vi "运维调试_氨氮.vi"() -> ()   [LabVIEW 2016, in "氨氮.lvlib"]
uses:
  <vilib>/Platform/TimedLoop/XDataNode/timing_clust.ctl
  <vilib>/Platform/TimedLoop/XDataNode/nitl_modes.ctl
  <vilib>/Platform/TimedLoop/XDataNode/wakeup.ctl
  <vilib>/Utility/miscctls.llb/LVPointTypeDef.ctl
  <vilib>/Platform/TimedLoop/XDataNode/XDataNode.xnode
  <vilib>/Platform/TimedLoop/XDataNode/XDNodeRunTimeDep.lvlib
  <vilib>/Utility/config.llb/NI_LVConfig.lvlib
panel:
  in  "氨氮自动测试量程配置":T1
  out "ADC":sgl
  out "温度2":sgl
  out "温度1":sgl
  out "固件版本号":string
  in  "数组":string[](array[string])
  in  "备用系数写入":bool
  in  "备用系数读取":bool
  in  "备用系数":T2
  in  "量程切换阈值写入":bool
  in  "量程切换阈值读取":bool
  in  "量程切换阈值":cluster{"阈值":dbl, "标液浓度":dbl}
  in  "参数下拉列表":enum16{"氨氮", "总磷"}(ring)
  in  "量程下拉列表":enum16{"低量程", "高量程"}(ring)
  in  "测量模式下拉列表":enum16{"水样测量", "空白核查", "跨度核查", "标样核查", "加标回收"}(ring)
  in  "公式":cluster{"X^2":dbl, "X":dbl, "b":dbl}
  in  "写公式":bool
  in  "读公式":bool
  in  "精度":dbl=4.0
  in  "样品5 F0":dbl
  in  "样品5 F1":dbl
  in  "样品4 F1":dbl
  in  "样品4 F0":dbl
  in  "样品3 F0":dbl
  in  "样品3 F1":dbl
  in  "样品2 F0":dbl
  in  "样品2 F1":dbl
  in  "样品1 F1":dbl
  in  "样品1 F0":dbl
  in  "method":u16(ring) items=["最小二乘", "最小绝对残差", "Bisquare"]
  in  "模型":enum32{"线性", "多项式"}(ring)
  out "r^2":dbl format="%.7g"
  out "拟合公式":string
  in  "样品2启用":bool
  in  "样品5启用":bool
  in  "样品4启用":bool
  in  "样品3启用":bool
  in  "样品1启用":bool
  in  "标液浓度5":dbl
  out "测量吸光度5":dbl
  in  "标液浓度4":dbl
  out "测量吸光度4":dbl
  in  "标液浓度3":dbl
  out "测量吸光度3":dbl
  in  "标液浓度2":dbl
  out "测量吸光度2":dbl
  out "测量吸光度1":dbl
  in  "标液浓度1":dbl
  out "XY图":cluster{"X Values":dbl[], "Y Values":dbl[]}[](graph)
  in  "返回":bool
  in  "设置":bool
  out "序列号":string="序列号"
  out "氨氮测量数据":T3(xcontrol)
  out "集成报警信息":string
  out "设置值":dbl
  out "定时启动":bool
  out "总磷总氮运行状态":T4(xcontrol)
  in  "停止":bool
  in  "手动启动":bool
  in  "单步测试":bool
  in  "总磷氨氮调试":u16[](xcontrol)
  out "F3":sgl format="%#.6f"
  out "F2":sgl format="%#.6f"
  out "F1":sgl format="%#.6f"
  out "F0":sgl format="%#.6f"
  out "多列列表框":i32(listbox)
  # "COM7"
  # "参数设置"
  # "标液浓度"
  # "F0"
  # "F1"
  # "吸光值显示"
  # "样品一"
  # "辅\n助\n计\n算\n区"
  # "样品二"
  # "样品三"
  # "样品四"
  # "样品五"
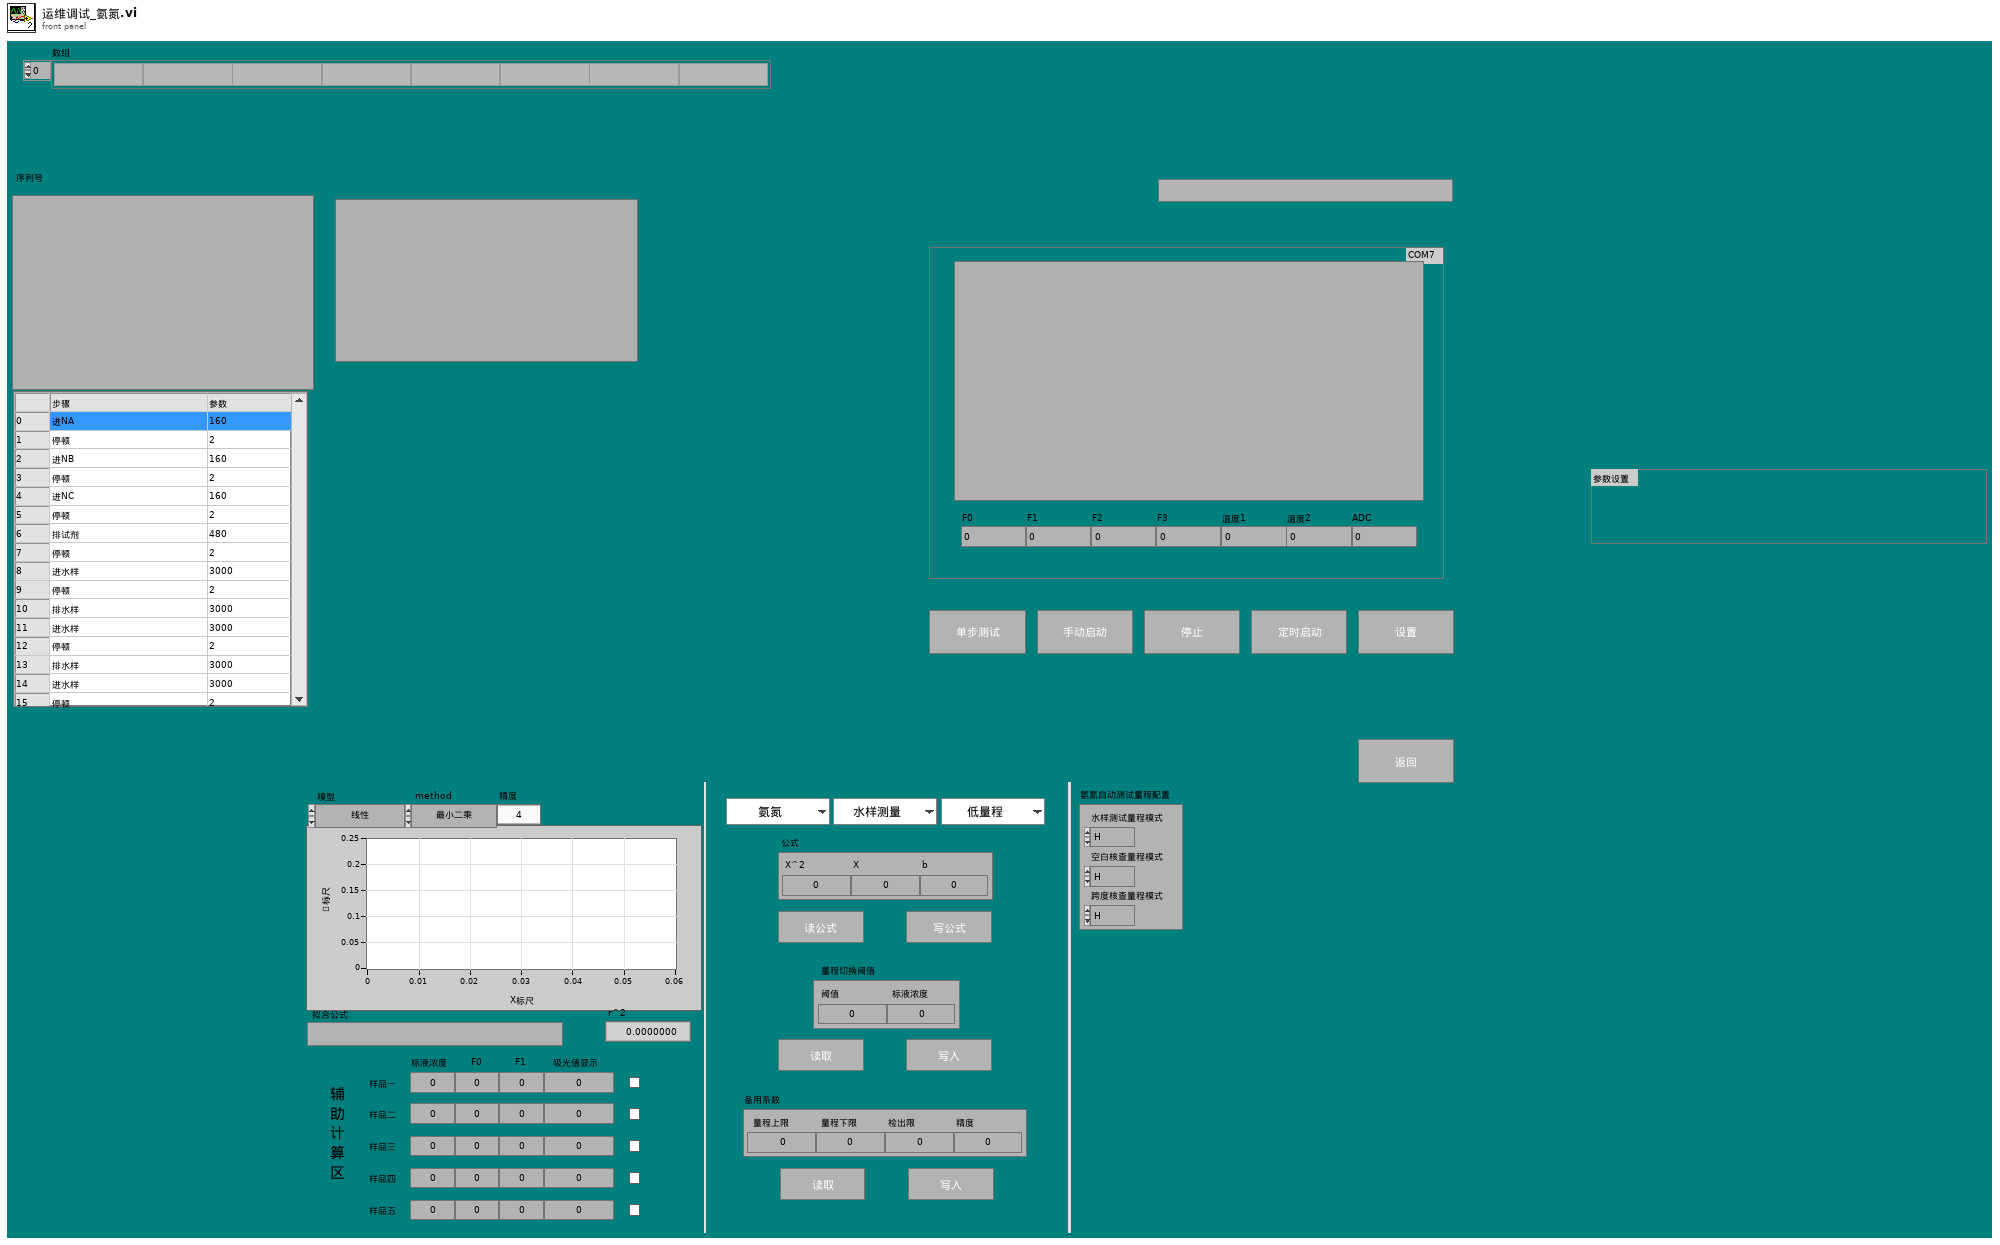
[diagram p1: front panel]
types:
  T1 = cluster{"水样测试量程模式":enum16{"H", "L", "AUTO"}, "空白核查量程模式":enum16{"H", "L", "AUTO"}, "跨度核查量程模式":enum16{"H", "L", "AUTO"}}
  T2 = cluster{"量程上限":dbl, "量程下限":dbl, "检出限":dbl, "精度":dbl}
  T3 = cluster{"flowid":u16, "测量精度":u16, "测量数据区":cluster{"因子编码":u32, "单位":u16, "标样参考值":sgl, "水样数据时间":timestamp, "水样实测值":sgl, "水样数据标识":string, "标样数据时间":timestamp, "标样实测值":sgl, "标样数据标识":string, "空白数据时间":timestamp, "空白实测值":sgl, "空白数据标识":string, "零点核查数据时间":timestamp, "零点核查实测值":sgl, "零点核查数据标识":string, "跨度核查数据时间":timestamp, "跨度核查实测值":sgl, "跨度核查数据标识":string, "加标回收数据时间":timestamp, "加标回收实测值":sgl, "加标回收数据标识":string, "平行样数据时间":timestamp, "平行样实测值":sgl, "平行样数据标识":string}}
  T4 = cluster{"系统时间":timestamp, "工作状态":enum16{"空闲", "水样测试", "标样核查", "零点核查", "跨度核查", "空白测试", "平行样测试", "加标回收", "空白校准", "标样校准", "初始化（清洗）"}, "测量模式":enum16{"待机", "连续模式", "周期模式", "定点模式", "受控模式", "手动模式"}, "告警代码":enum16{"无告警", "缺试剂告警", "缺水样告警", "缺蒸馏水告警", "缺标液告警", "仪表漏液告警", "标定异常告警", "超量程告警", "加热异常", "低试剂预警", "超上限告警", "超下限告警", "仪表内部其他异常", "滴定异常告警", "电极异常告警", "量程切换告警", "参数设置告警", "PH电极电位异常", "电导率电极异常", "浊度光度异常", "溶解氧电极异常", "溶解氧光强异常", "温度异常告警", "PH异常告警", "溶解氧异常告警", "电导率异常告警", "浊度异常告警", "叶绿素异常告警", "藻密度异常告警", "蓝绿藻异常告警", "ORP异常告警", "氨氮异常告警", "清洁刷异常告警", "SD卡异常告警", "蓝牙异常告警", "Wifi异常告警", "流程异常告警"}, "故障代码":enum16{"无故障", "电机故障", "温度故障", "通讯故障", "滴定故障"}, "日志代码":u16, "软件版本":u16, "F0":sgl, "F1":sgl, "F2":sgl, "F3":sgl, "T":sgl, "H":sgl, "id":u16, "flowid":u16, "量程":u16, "总磷控温温度1":sgl, "营养盐控温温度2":sgl, "ADC":sgl}
  T5 = enum16{"待机", "启动氨氮", "氨氮测量中", "启动总磷", "总磷测量中", "延时"}
  T6 = typedef "LVPointTypeDef.ctl" = cluster{"Horizontal":i16, "Vertical":i16}
  T7 = cluster{"因子编码":u32, "单位":u16, "标样参考值":sgl, "水样数据时间":timestamp, "水样实测值":sgl, "水样数据标识":string, "标样数据时间":timestamp, "标样实测值":sgl, "标样数据标识":string, "空白数据时间":timestamp, "空白实测值":sgl, "空白数据标识":string, "零点核查数据时间":timestamp, "零点核查实测值":sgl, "零点核查数据标识":string, "跨度核查数据时间":timestamp, "跨度核查实测值":sgl, "跨度核查数据标识":string, "加标回收数据时间":timestamp, "加标回收实测值":sgl, "加标回收数据标识":string, "平行样数据时间":timestamp, "平行样实测值":sgl, "平行样数据标识":string}
  T8 = enum16{"空闲", "水样测试", "标样核查", "零点核查", "跨度核查", "空白测试", "平行样测试", "加标回收", "空白校准", "标样校准", "初始化（清洗）"}
  T9 = cluster{"启动模式":enum16{"标液测量", "水样测量", "零液测量", "盲样测量", "加标回收"}, "启动参数":u16, "量程":enum16{"低量程", "高量程"}}
  T10 = cluster{"时间标识":timestamp, "设备":string, "日志信息":string, "流程参数":string}
  T11 = cluster{"时间标识":timestamp, "设备":string, "日志信息":string}
  T12 = enum16{"无告警", "缺试剂告警", "缺水样告警", "缺蒸馏水告警", "缺标液告警", "仪表漏液告警", "标定异常告警", "超量程告警", "加热异常", "低试剂预警", "超上限告警", "超下限告警", "仪表内部其他异常", "滴定异常告警", "电极异常告警", "量程切换告警", "参数设置告警", "PH电极电位异常", "电导率电极异常", "浊度光度异常", "溶解氧电极异常", "溶解氧光强异常", "温度异常告警", "PH异常告警", "溶解氧异常告警", "电导率异常告警", "浊度异常告警", "叶绿素异常告警", "藻密度异常告警", "蓝绿藻异常告警", "ORP异常告警", "氨氮异常告警", "清洁刷异常告警", "SD卡异常告警", "蓝牙异常告警", "Wifi异常告警", "流程异常告警"}
  T13 = typedef "LVRowAndColumnUnsignedTypeDef.ctl" = cluster{"Row":u32, "Column":u32}
  T14 = typedef "XDNodeRunTimeDep.lvlib/timing_clust.ctl" = cluster{"Expected End [f-1]":u64, "Actual End [f-1]":u64, "Finished Late? [f-1]":bool, "Expected End [i-1]":u64, "Actual End [i-1]":u64, "Finished Late? [i-1]":bool, "Expected Start [i]":u64, "Actual Start [i]":u64, "Expected Start [f]":u64, "Actual Start [f]":u64, "Source Name":string, "Structure Name":string, "Period":i64, "Deadline":i64, "Offset":i64, "Start":i64, "Priority":i32, "Timeout":i32, "Mode":T15, "Wakeup Reason":T16, "Error":errorcluster, "Source Type":string, "Secondary Source Type":string, "Global End Time":u64, "Global Start Time":u64, "Frame Duration":u64, "Iteration Duration":u64, "Assigned CPU":i32, "I/O Scan Engine Mode":u32}
  T15 = typedef "XDNodeRunTimeDep.lvlib/nitl_modes.ctl" = enum32{"No Change", "Process missed periods, maintain original phase", "Discard missed periods, maintain original phase", "Process missed periods, ignore original phase", "Discard missed periods, ignore original phase"}
  T16 = typedef "XDNodeRunTimeDep.lvlib/wakeup.ctl" = enum32{"Normal", "Aborted", "Asynchronous wakeup", "Timing source error", "Timed loop error", "Timeout"}
  T17 = cluster{"站号":u16, "量程切换":enum32{"H", "L", "AUTO"}, "控制命令":enum16{"启动测量", "标样核查", "零点核查", "跨度核查", "空白测试", "平行样测试", "加标回收", "空白校准", "标样校准", "初始化（清洗）", "停止测试", "仪器重启", "校时", "模式设置", "测量间隔设置", "盲样测试"}, "模式设置":enum16{"待机", "连续模式", "周期模式", "定点模式", "受控模式", "手动模式"}, "测量间隔":u16}
  T18 = typedef "NI_LVConfig.lvlib/Config Data RefNum.ctl" = refnum<k1>
  T19 = cluster{"站号":u16, "量程切换":enum32{"H", "L", "AUTO"}, "控制命令":enum16{"启动测量", "标样核查", "零点核查", "跨度核查", "空白测试", "平行样测试", "加标回收", "空白校准", "标样校准", "初始化（清洗）", "停止测试", "仪器重启", "校时", "模式设置", "测量间隔设置"}, "模式设置":enum16{"待机", "连续模式", "周期模式", "定点模式", "受控模式", "手动模式"}, "测量间隔":u16}
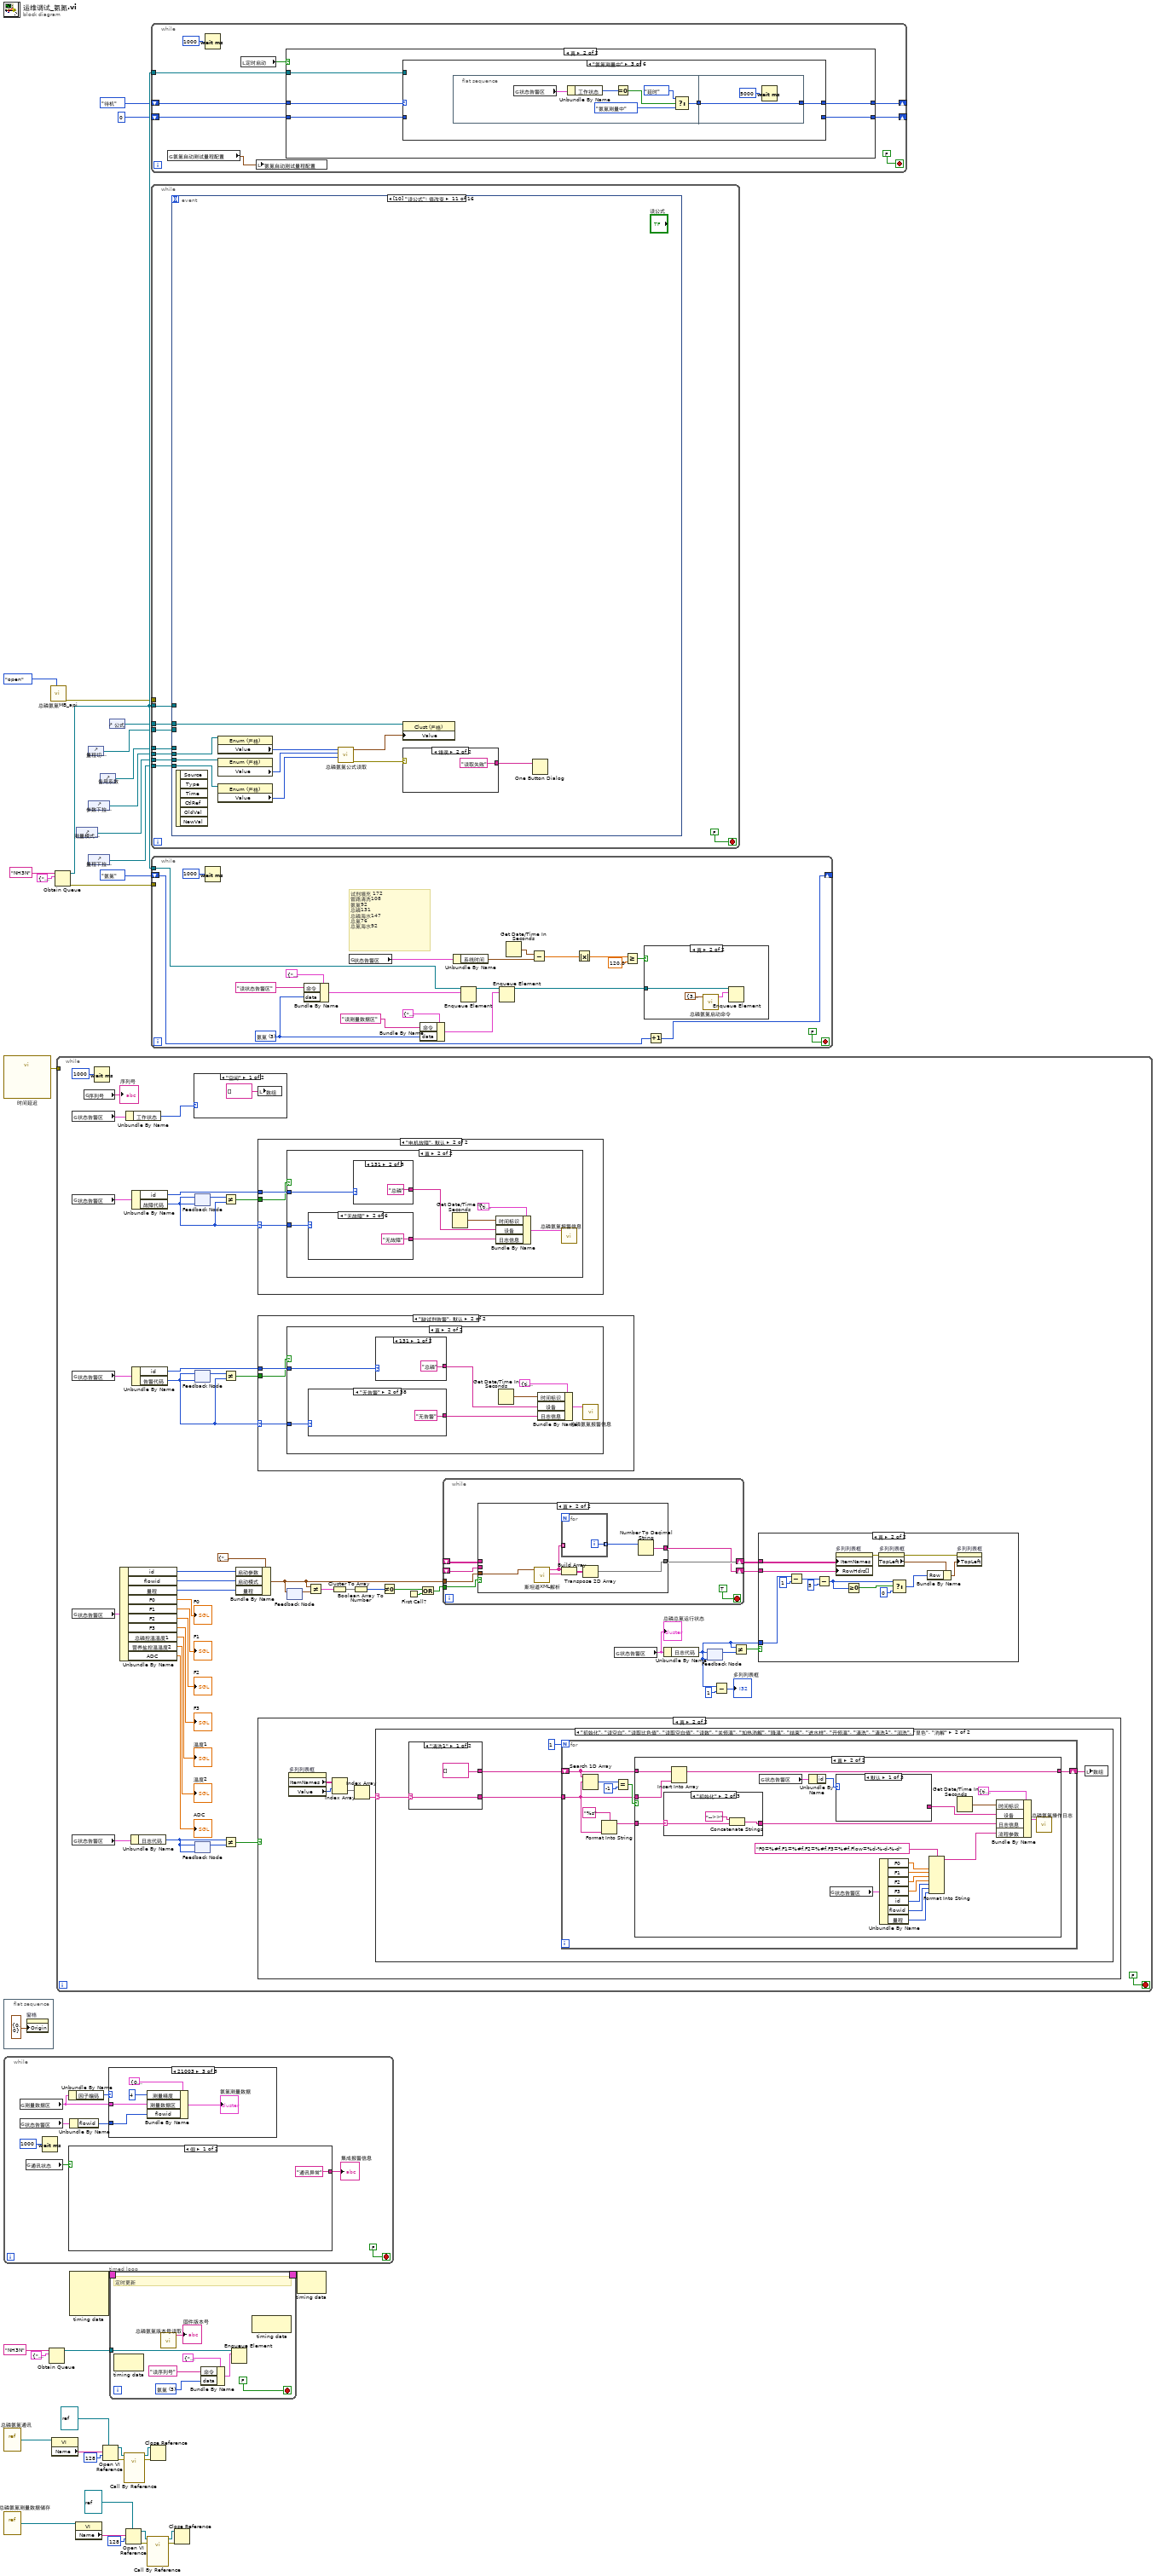
[diagram p0: block diagram]
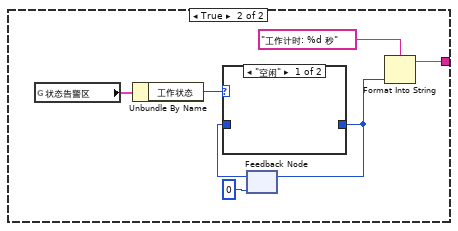
[diagram p2: hidden frame]
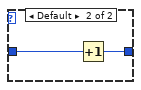
[diagram p3: hidden frame]
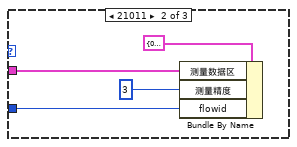
[diagram p5: hidden frame]
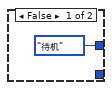
[diagram p6: hidden frame]
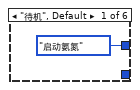
[diagram p7: hidden frame]
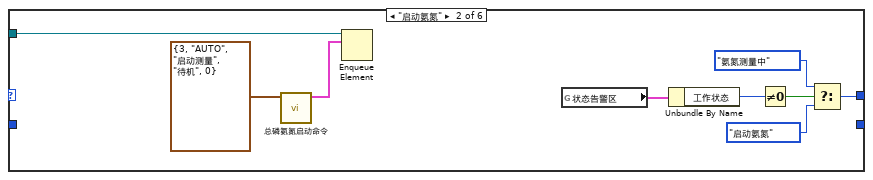
[diagram p8: hidden frame]
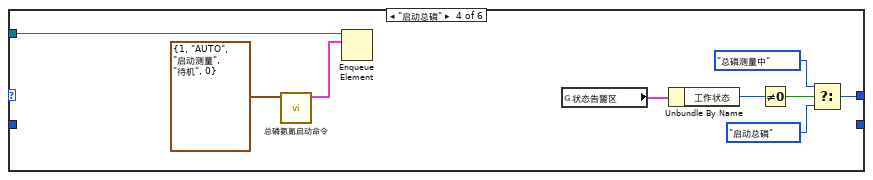
[diagram p9: hidden frame]
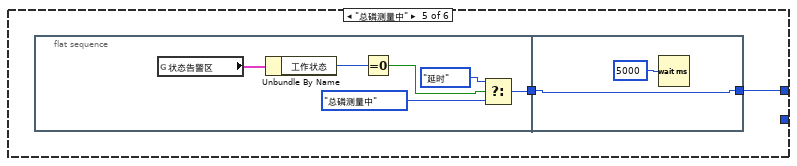
[diagram p10: hidden frame]
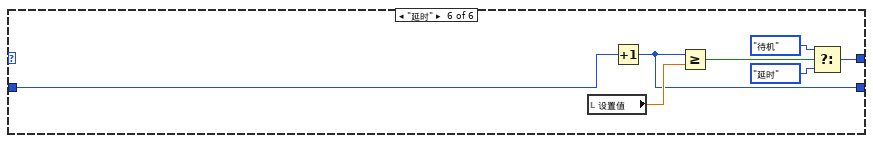
[diagram p11: hidden frame]
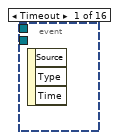
[diagram p12: hidden frame]
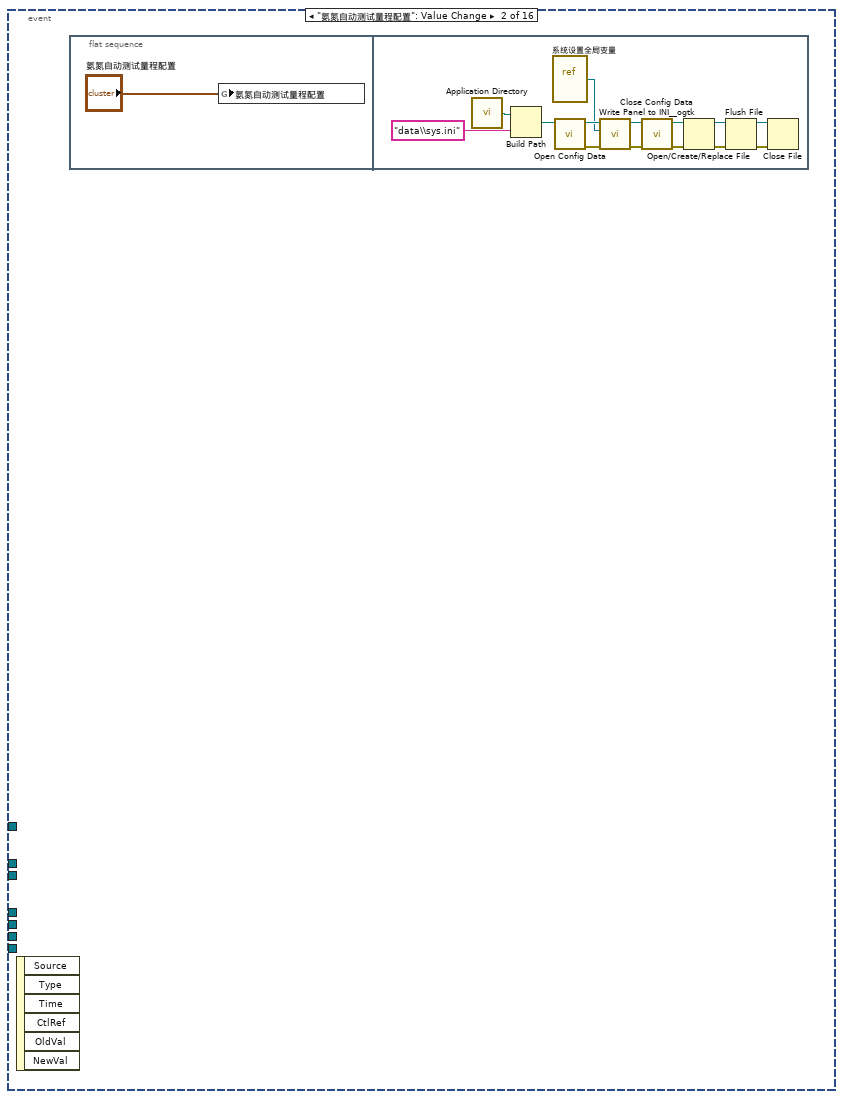
[diagram p13: hidden frame]
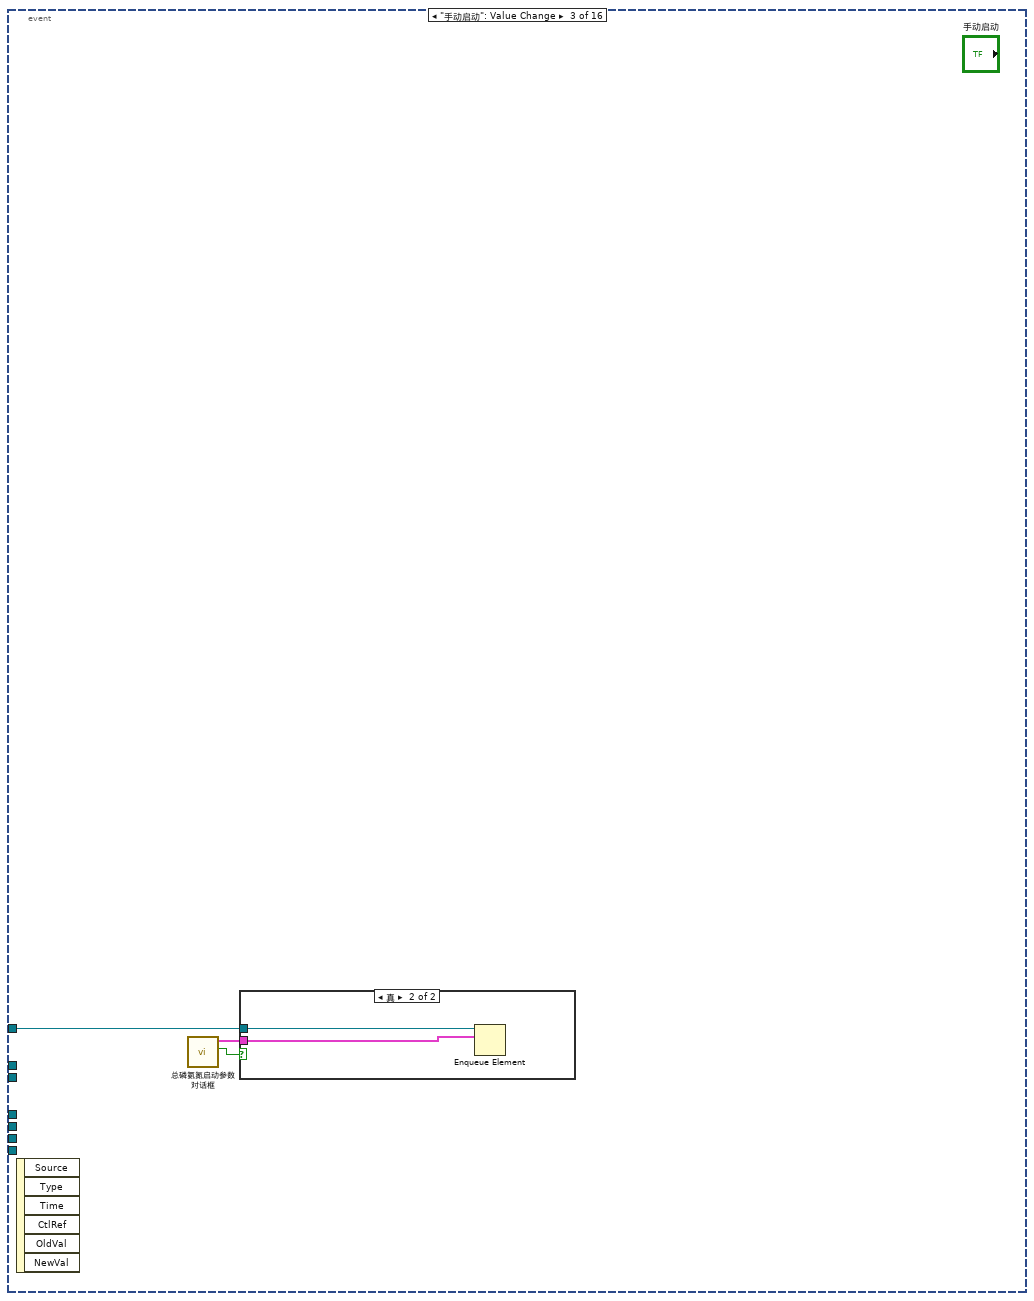
[diagram p14: hidden frame]
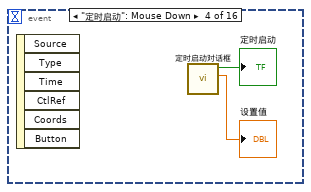
[diagram p16: hidden frame]
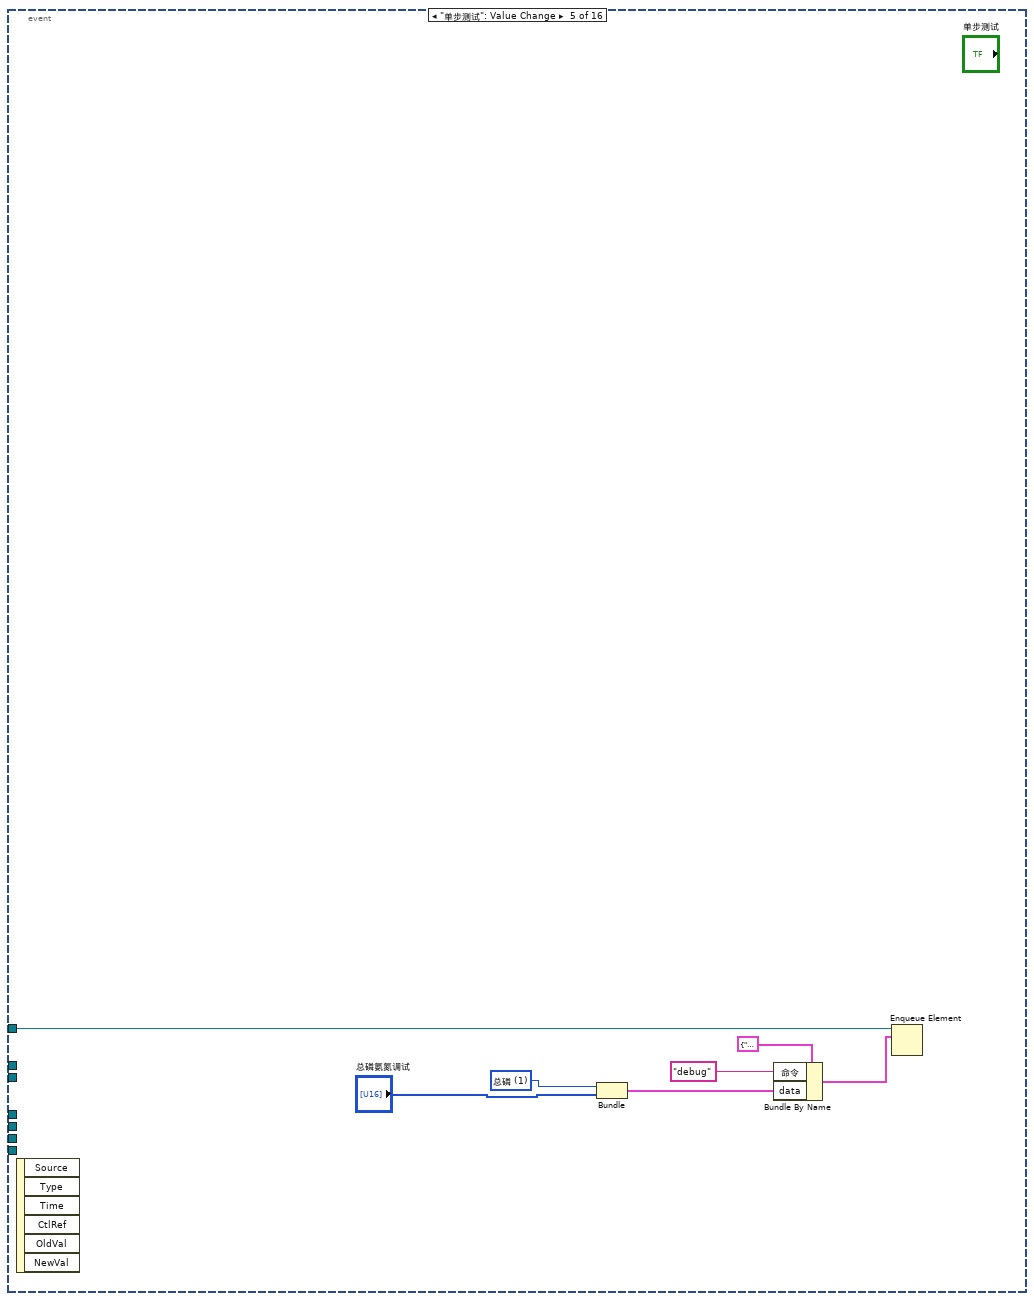
[diagram p17: hidden frame]
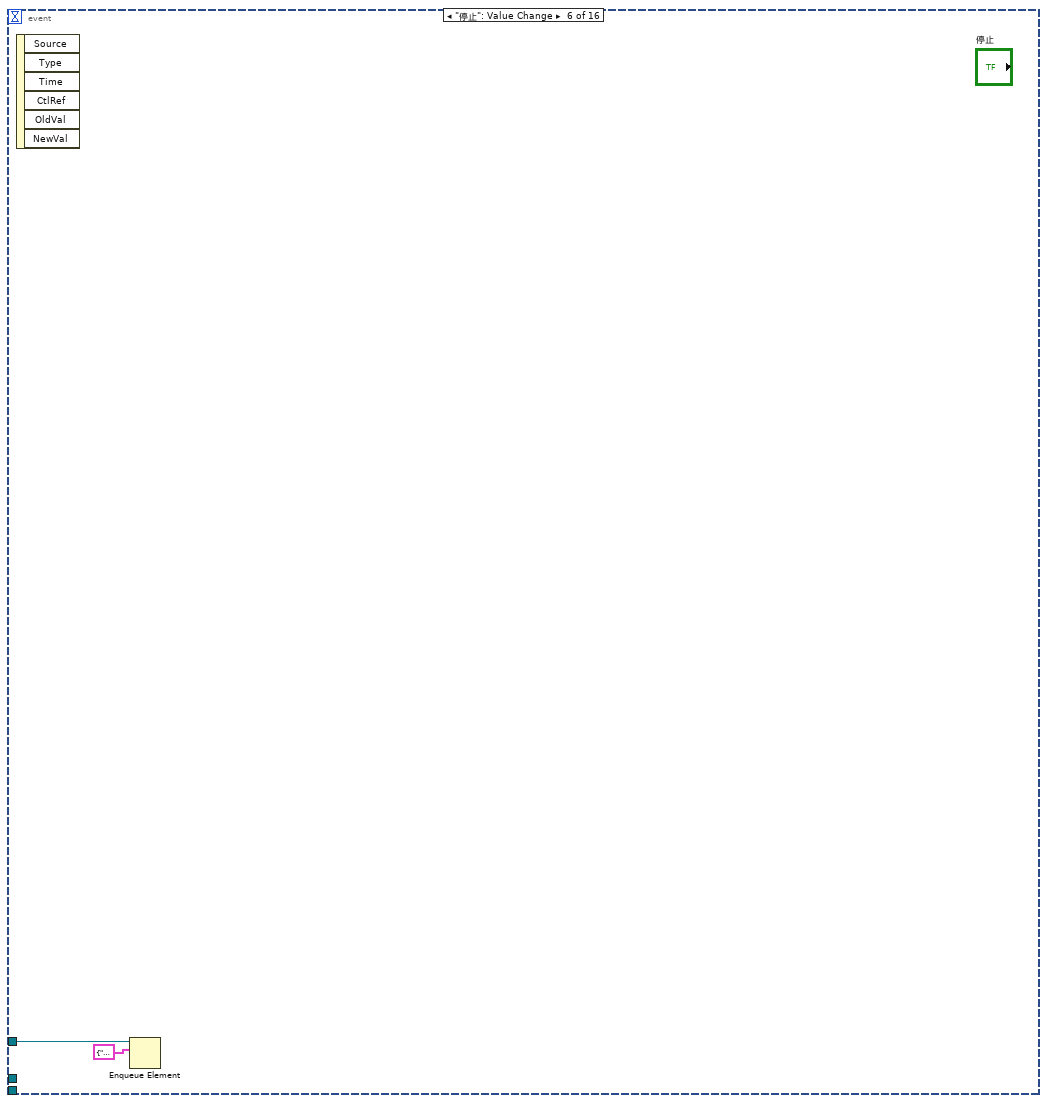
[diagram p18: hidden frame]
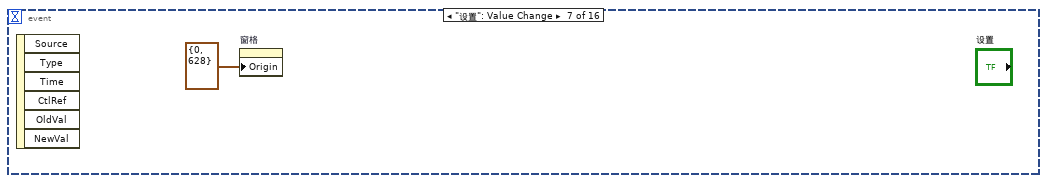
[diagram p19: hidden frame]
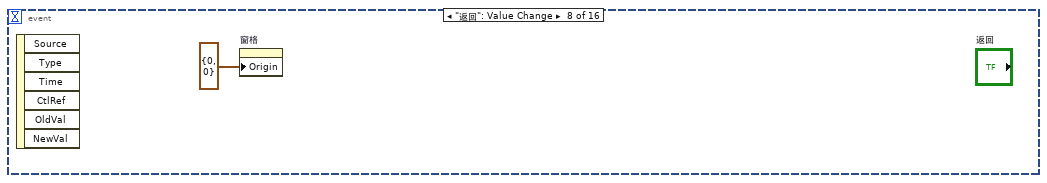
[diagram p20: hidden frame]
diagram:
  n1 = call "时间延迟"() -> ("error out"=w8:errorcluster)  [unwired: 11 in]
  n2 = flat-sequence {
    frame #0 {
      n3 = property on="窗格" class="Pane"("Origin"=T6 {"Horizontal"=0, "Vertical"=0} ("原点")) -> ()  [unwired: 2 in, 2 out]
    }
  }
  n4 = while {
    stop <- FALSE stop-if-true
    n5 = global read "VAR氨氮全局变量.vi" "测量数据区"() -> (w44:T7)
    n6 = global read "VAR氨氮全局变量.vi" "状态告警区"() -> (w40:T4)
    n7 = global read "VAR氨氮全局变量.vi" "通讯状态"() -> (w42:bool)
    n8 = Wait (ms)(milliseconds to wait=u32 1000 ("等待时间（毫秒）")) -> ()  [unwired: 1 out]
    n9 = Unbundle By Name(w44) -> ("因子编码"=w43:u32)
    n10 = case shown="假" w42 {
      tunnel: ["通讯异常" ("集成报警信息") w48] -> w41
      frame False {
      }
      frame True {
        n11 = global read "VAR氨氮全局变量.vi" "状态告警区"() -> (w54:T4)
        n12 = Unbundle By Name(w54) -> ("工作状态"=w53:T8)
        n13 = feedback #1(0) -> (w51:i32)
        n14 = case shown="\"空闲\"" w53 {
          tunnel: w51 -> [_ w56]
          tunnel: [_ w55] -> w49
          frame "空闲" {
          }
          frame Default {
            n15 = Increment(x=w56) -> (x+1=w55:i32)
          }
        }
        n16 = feedback-in #1(w49) -> ()
        n17 = Format Into String(format string="工作计时: %d 秒" ("格式字符串"), w49) -> (resulting string=w48:string)  [unwired: 2 in, 1 out]
      }
    }
    "集成报警信息" <- w41
    n18 = Unbundle By Name(w40) -> ("flowid"=w39:u16)
    n19 = case shown="21003" w43 {
      tunnel: w44 -> [_ w60 w65]
      tunnel: w39 -> [_ w58 w63]
      frame Default {
      }
      frame 21011 {
        n20 = Bundle By Name(cluster=T3 {"flowid"=0, "测量精度"=0, "测量数据区"={"因子编码"=0, "单位"=0, "标样参考值"=0.0, "水样数据时间"=timestamp(0 s since 1904-01-01), "水样实测值"=0.0, "水样数据标识"="", "标样数据时间"=timestamp(0 s since 1904-01-01), "标样实测值"=0.0, "标样数据标识"="", "空白数据时间"=timestamp(0 s since 1904-01-01), "空白实测值"=0.0, "空白数据标识"="", "零点核查数据时间"=timestamp(0 s since 1904-01-01), "零点核查实测值"=0.0, "零点核查数据标识"="", "跨度核查数据时间"=timestamp(0 s since 1904-01-01), "跨度核查实测值"=0.0, "跨度核查数据标识"="", "加标回收数据时间"=timestamp(0 s since 1904-01-01), "加标回收实测值"=0.0, "加标回收数据标识"="", "平行样数据时间"=timestamp(0 s since 1904-01-01), "平行样实测值"=0.0, "平行样数据标识"=""}} ("氨氮测量数据"), "测量数据区"=w60, "测量精度"=u16 3, "flowid"=w58) -> ()  [unwired: 1 out]
      }
      frame 21003 {
        n21 = Bundle By Name(cluster=T3 {"flowid"=0, "测量精度"=0, "测量数据区"={"因子编码"=0, "单位"=0, "标样参考值"=0.0, "水样数据时间"=timestamp(0 s since 1904-01-01), "水样实测值"=0.0, "水样数据标识"="", "标样数据时间"=timestamp(0 s since 1904-01-01), "标样实测值"=0.0, "标样数据标识"="", "空白数据时间"=timestamp(0 s since 1904-01-01), "空白实测值"=0.0, "空白数据标识"="", "零点核查数据时间"=timestamp(0 s since 1904-01-01), "零点核查实测值"=0.0, "零点核查数据标识"="", "跨度核查数据时间"=timestamp(0 s since 1904-01-01), "跨度核查实测值"=0.0, "跨度核查数据标识"="", "加标回收数据时间"=timestamp(0 s since 1904-01-01), "加标回收实测值"=0.0, "加标回收数据标识"="", "平行样数据时间"=timestamp(0 s since 1904-01-01), "平行样实测值"=0.0, "平行样数据标识"=""}} ("氨氮测量数据"), "测量精度"=u16 4, "测量数据区"=w65, "flowid"=w63) -> (→"氨氮测量数据":T3)
      }
    }
  }
  n22 = vi-ref "总磷氨氮通讯.vi"() -> (w31:refnum<vi>)
  n23 = vi-ref "总磷氨氮测量数据储存.vi"() -> (w23:refnum<vi>)
  n24 = Obtain Queue(name (unnamed)="NH3N" ("名称（未命名）"), element data type=cluster{"命令":string, "data":variant} {"命令"="", "data"=variant}) -> (queue out=w1:refnum<queue>)  [unwired: 3 in, 2 out]
  n25 = call "总磷氨氮MB_api.vi"("STEP"=enum16{"open", "read", "write", "close"}."open") -> ("error out"=w7:errorcluster)  [unwired: 8 in, 2 out]
  n26 = property class="VI"(reference=w31) -> ("Name"=w30:string)  [unwired: 1 in, 2 out]
  n27 = Obtain Queue(name (unnamed)="NH3N" ("名称（未命名）"), element data type=cluster{"命令":string, "data":variant} {"命令"="", "data"=variant}) -> (queue out=w34:refnum<queue>, error out=w35:errorcluster)  [unwired: 3 in, 1 out]
  n28 = while {
    tunnel: w8 -> [_]
    stop <- FALSE stop-if-true
    n29 = global read "VAR氨氮全局变量.vi" "状态告警区"() -> (w77:T4)
    n30 = global read "VAR氨氮全局变量.vi" "状态告警区"() -> (w82:T4)
    n31 = global read "VAR氨氮全局变量.vi" "状态告警区"() -> (w87:T4)
    n32 = global read "VAR氨氮全局变量.vi" "状态告警区"() -> (w99:T4)
    n33 = global read "VAR氨氮全局变量.vi" "状态告警区"() -> (w74:T4)
    n34 = global read "VAR氨氮全局变量.vi" "序列号"() -> (→"序列号":string)
    n35 = Wait (ms)(milliseconds to wait=u32 1000 ("等待时间（毫秒）")) -> ()  [unwired: 1 out]
    n36 = Unbundle By Name(w99) -> ("id"=w96:u16, "flowid"=w98:u16, "量程"=w97:u16, "F0"=→"F0":sgl, "F1"=→"F1":sgl, "F2"=→"F2":sgl, "F3"=→"F3":sgl, "总磷控温温度1"=→"温度1":sgl, "营养盐控温温度2"=→"温度2":sgl, "ADC"=→"ADC":sgl)
    n37 = Unbundle By Name(w77) -> ("工作状态"=w76:T8)
    n38 = Unbundle By Name(w74) -> ("日志代码"=w73:u16)
    n39 = Unbundle By Name(w82) -> ("id"=w81:u16, "故障代码"=w78:enum16{"无故障", "电机故障", "温度故障", "通讯故障", "滴定故障"})
    n40 = Unbundle By Name(w87) -> ("id"=w86:u16, "告警代码"=w83:T12)
    n41 = case shown="\"空闲\"" w76 {
      frame "空闲" {
        n42 = local write "数组"(string[] [] ("数组")) -> ()
      }
      frame "水样测试", Default {
      }
    }
    n43 = feedback #2(w78) -> (w79:enum16{"无故障", "电机故障", "温度故障", "通讯故障", "滴定故障"})
    n44 = feedback-in #2(w78) -> ()
    n45 = feedback #3(w83) -> (w84:T12)
    n46 = feedback-in #3(w83) -> ()
    n47 = feedback #4(w73) -> (w75:u16)
    n48 = feedback-in #4(w73) -> ()
    n49 = Not Equal?(x=w79, y=w78) -> (x != y?=w80:bool)
    n50 = Not Equal?(x=w84, y=w83) -> (x != y?=w85:bool)
    n51 = Not Equal?(x=w73, y=w75) -> (x != y?=w72:bool)
    n52 = Bundle By Name(cluster=T9 {"启动模式"=enum."加标回收", "启动参数"=1, "量程"=enum."低量程"} ("参数簇"), "启动参数"=w96, "启动模式"=w98, "量程"=w97) -> (w89:T9)
    n53 = case shown="\"电机故障\", 默认" w78 {
      selector: w78 -> [_ w167]
      tunnel: w81 -> [_ w168]
      tunnel: w80 -> [_ w166]
      frame "无故障" {
      }
      frame "电机故障", Default {
        n54 = case shown="真" w166 {
          tunnel: w168 -> [_ w175]
          tunnel: w167 -> [_ w170]
          frame False {
          }
          frame True {
            n55 = case shown="\"无故障\"" w170 {
              selector: w170 -> [w177 _ _ _ _ _]
              tunnel: [w176 "无故障" "电机故障" "温度故障" "通讯故障" "滴定故障"] -> w169
              frame Default {
                n56 = Format Into String(format string="%d" ("格式字符串"), initial string="未知" ("工作状态"), w177) -> (resulting string=w176:string)  [unwired: 1 in, 1 out]
              }
              frame "无故障" {
              }
              frame "电机故障" {
              }
              frame "温度故障" {
              }
              frame "通讯故障" {
              }
              frame "滴定故障" {
              }
            }
            n57 = case shown="131" w175 {
              tunnel: [_ "总磷" ("table输入") "氨氮" ("table输入")] -> w171
              frame Default {
              }
              frame 131 {
              }
              frame 92 {
              }
            }
            n58 = Get Date/Time In Seconds() -> (seconds since 1Jan1904=w172:timestamp)
            n59 = Bundle By Name(cluster=T11 {"时间标识"=timestamp(0 s since 1904-01-01), "设备"="", "日志信息"=""} ("data in"), "时间标识"=w172, "设备"=w171, "日志信息"=w169) -> (w173:T11)
            n60 = call "总磷氨氮报警信息.vi"("data in"=w173) -> ()  [unwired: 11 in]
          }
        }
      }
    }
    n61 = case shown="\"缺试剂告警\", 默认" w83 {
      selector: w83 -> [_ w188]
      tunnel: w86 -> [_ w189]
      tunnel: w85 -> [_ w187]
      frame "无告警" {
      }
      frame "缺试剂告警", Default {
        n62 = case shown="真" w187 {
          tunnel: w189 -> [_ w196]
          tunnel: w188 -> [_ w190]
          frame False {
          }
          frame True {
            n63 = case shown="\"无告警\"" w190 {
              selector: w190 -> [w198 _ _ _ _ _ _ _ _ _ _ _ _ _ _ _ _ _ _ _ _ _ _ _ _ _ _ _ _ _ _ _ _ _ _ _ _ _]
              tunnel: [w197 "无告警" "缺试剂告警" "缺水样告警" "缺蒸馏水告警" "缺标液告警" "仪表漏液告警" "标定异常告警" "超量程告警" "加热异常" "低试剂预警" "超上限告警" "超下限告警" "仪表内部其他异常" "滴定异常告警" "电极异常告警" "量程切换告警" "参数设置告警" "PH电极电位异常" "电导率电极异常" "浊度光度异常" "溶解氧电极异常" "溶解氧光强异常" "温度异常告警" "PH异常告警" "溶解氧异常告警" "电导率异常告警" "浊度异常告警" "叶绿素异常告警" "藻密度异常告警" "蓝绿藻异常告警" "ORP异常告警" "氨氮异常告警" "清洁刷异常告警" "SD卡异常告警" "蓝牙异常告警" "WiFi异常告警" "流程异常告警"] -> w191
              frame Default {
                n64 = Format Into String(format string="%d" ("格式字符串"), initial string="未知" ("工作状态"), w198) -> (resulting string=w197:string)  [unwired: 1 in, 1 out]
              }
              frame "无告警" {
              }
              frame "缺试剂告警" {
              }
              frame "缺水样告警" {
              }
              frame "缺蒸馏水告警" {
              }
              frame "缺标液告警" {
              }
              frame "仪表漏液告警" {
              }
              frame "标定异常告警" {
              }
              frame "超量程告警" {
              }
              frame "加热异常" {
              }
              frame "低试剂预警" {
              }
              frame "超上限告警" {
              }
              frame "超下限告警" {
              }
              frame "仪表内部其他异常" {
              }
              frame "滴定异常告警" {
              }
              frame "电极异常告警" {
              }
              frame "量程切换告警" {
              }
              frame "参数设置告警" {
              }
              frame "PH电极电位异常" {
              }
              frame "电导率电极异常" {
              }
              frame "浊度光度异常" {
              }
              frame "溶解氧电极异常" {
              }
              frame "溶解氧光强异常" {
              }
              frame "温度异常告警" {
              }
              frame "PH异常告警" {
              }
              frame "溶解氧异常告警" {
              }
              frame "电导率异常告警" {
              }
              frame "浊度异常告警" {
              }
              frame "叶绿素异常告警" {
              }
              frame "藻密度异常告警" {
              }
              frame "蓝绿藻异常告警" {
              }
              frame "ORP异常告警" {
              }
              frame "氨氮异常告警" {
              }
              frame "清洁刷异常告警" {
              }
              frame "SD卡异常告警" {
              }
              frame "蓝牙异常告警" {
              }
              frame "Wifi异常告警" {
              }
              frame "流程异常告警" {
              }
            }
            n65 = case shown="131" w196 {
              tunnel: ["总磷" ("table输入") "氨氮" ("table输入")] -> w192
              frame 131 {
              }
              frame 92, Default {
              }
            }
            n66 = Get Date/Time In Seconds() -> (seconds since 1Jan1904=w193:timestamp)
            n67 = Bundle By Name(cluster=T11 {"时间标识"=timestamp(0 s since 1904-01-01), "设备"="", "日志信息"=""} ("data in"), "时间标识"=w193, "设备"=w192, "日志信息"=w191) -> (w194:T11)
            n68 = call "总磷氨氮报警信息.vi"("data in"=w194) -> ()  [unwired: 11 in]
          }
        }
      }
    }
    n69 = case shown="真" w72 {
      frame False {
      }
      frame True {
        n70 = property on="多列列表框" class="MCListbox (严格)"() -> ("ItemNames"=w116:string[][], "Value"=w117:i32)  [unwired: 2 in, 2 out]
        n71 = Index Array(array=w116, index (row)=w117) -> (element=w115:string[])  [unwired: 1 in]
        n72 = Index Array(array=w115) -> (element=w114:string)  [unwired: 1 in]
        n73 = case shown="\"初始化\", \"读空白\", \"读取比色值\", \"读取空白值\", \"读数\", \"关恒温\", \"加热消解\", \"降温\", \"结束\", \"进水样\", \"开恒温\", \"清洗\", \"清洗1\", \"润洗\", \"显色\", \"消解\"" w114 {
          selector: w114 -> [_ w120]
          frame Default {
          }
          frame "初始化", "读空白", "读取比色值", "读取空白值", "读数", "关恒温", "加热消解", "降温", "结束", "进水样", "开恒温", "清洗", "清洗1", "润洗", "显色", "消解" {
            n74 = case shown="\"清洗1\"" w120 {
              selector: w120 -> [w124 w126]
              tunnel: [w124 w126] -> w119
              tunnel: [string[] [] ("数组") "数组"] -> w118
              frame "清洗1" {
              }
              frame Default {
              }
            }
            n75 = for {
              N: 1 -> [_]
              tunnel: w119 -> [w128]
              shift-right: [w127] -> w121
              shift-left: w118 -> [w129]
              n76 = Search 1D Array(1D array=w129, element=w128) -> (index of element=w132:i32)  [unwired: 1 in]
              n77 = Format Into String(format string="%s" ("格式字符串"), w128) -> (resulting string=w133:string)  [unwired: 2 in, 1 out]
              n78 = Equal?(x=w132, y=-1) -> (x = y?=w130:bool)
              n79 = case shown="真" w130 {
                tunnel: w133 -> [_ w137]
                tunnel: w129 -> [w135 w141]
                tunnel: w128 -> [_ w140]
                tunnel: [w135 w139] -> w127
                frame False {
                }
                frame True {
                  n80 = case shown="\"初始化\"" w137 {
                    selector: w137 -> [w157 w160 w163]
                    tunnel: [w157 w159 w162] -> w136
                    frame Default {
                    }
                    frame "初始化" {
                      n81 = Concatenate Strings("-->>" ("字符串"), w160) -> (w159:string)
                    }
                    frame "结束" {
                      n82 = Concatenate Strings("-->>" ("字符串"), w163) -> (w162:string)
                    }
                  }
                  n83 = Insert Into Array(array=w141, new element=w140) -> (w139:string[])  [unwired: 1 in]
                  n84 = global read "VAR氨氮全局变量.vi" "状态告警区"() -> (w156:T4)
                  n85 = Unbundle By Name(w156) -> ("id"=w155:u16)
                  n86 = global read "VAR氨氮全局变量.vi" "状态告警区"() -> (w151:T4)
                  n87 = case shown="默认" w155 {
                    tunnel: [_ "总磷" ("table输入") "氨氮" ("table输入")] -> w153
                    frame Default {
                    }
                    frame 131 {
                    }
                    frame 92 {
                    }
                  }
                  n88 = Unbundle By Name(w151) -> ("F0"=w148:sgl, "F1"=w147:sgl, "F2"=w146:sgl, "F3"=w145:sgl, "id"=w144:u16, "flowid"=w143:u16, "量程"=w142:u16)
                  n89 = Format Into String(format string="F0=%#f,F1=%#f,F2=%#f,F3=%#f,Flow=%d-%-d-%-d" ("格式字符串"), w148, w147, w146, w145, w144, w143, w142) -> (resulting string=w149:string)  [unwired: 2 in, 1 out]
                  n90 = Get Date/Time In Seconds() -> (seconds since 1Jan1904=w152:timestamp)
                  n91 = Bundle By Name(cluster=T10 {"时间标识"=timestamp(0 s since 1904-01-01), "设备"="", "日志信息"="", "流程参数"=""} ("data in"), "时间标识"=w152, "设备"=w153, "日志信息"=w136, "流程参数"=w149) -> (w154:T10)
                  n92 = call "总磷氨氮操作日志.vi"("data in"=w154) -> ()  [unwired: 11 in]
                }
              }
            }
            n93 = local write "数组"(w121) -> ()
          }
        }
      }
    }
    n94 = feedback #5() -> (w105:T9)  [unwired: 1 in]
    n95 = feedback-in #5(w89) -> ()
    n96 = Not Equal?(x=w89, y=w105) -> (x != y?=w106:cluster{"启动模式":bool, "启动参数":bool, "量程":bool})
    n97 = Cluster To Array(cluster=w106) -> (array=w107:bool[])
    n98 = Boolean Array To Number(Boolean array=w107) -> (number=w108:u32)
    n99 = Not Equal To 0?(x=w108) -> (x != 0?=w101:bool)
    n100 = First Call?() -> (First Call?: T/F=w102:bool)
    n101 = Or(x=w101, y=w102) -> (x .or. y?=w100:bool)
    n102 = while {
      tunnel: w100 -> [w246]
      tunnel: w89 -> [w245]
      shift-right: [w244] -> w104
      shift-left: _ -> [w240]
      shift-right: [w243] -> w103
      shift-left: _ -> [w241]
      stop <- TRUE stop-if-true
      n103 = case shown="真" w246 {
        tunnel: [w248 w255] -> w243
        tunnel: [w247 w254] -> w244
        tunnel: w245 -> [_ w249]
        tunnel: w241 -> [w248 _]
        tunnel: w240 -> [w247 _]
        frame False {
        }
        frame True {
          n104 = call "斯坦道XML解析.vi"("参数簇"=w249) -> ("步骤时间"=w250:string[], "步骤名"=w252:string[])  [unwired: 9 in]
          n105 = for {
            tunnel: w252 -> [_] mode=indexing
            tunnel: [w256] -> w253 mode=indexing
            i -> [w256]
          }
          n106 = Build Array(w252, w250) -> (w251:string[][])
          n107 = Transpose 2D Array(2D array=w251) -> (transposed array=w254:string[][])
          n108 = Number To Decimal String(number=w253) -> (decimal integer string=w255:string[])  [unwired: 1 in]
        }
      }
    }
    n109 = global read "VAR氨氮全局变量.vi" "状态告警区"() -> (w90:T4)
    "总磷总氮运行状态" <- w90
    n110 = Unbundle By Name(w90) -> ("日志代码"=w67:u16)
    n111 = feedback-in #6(w67) -> ()
    n112 = feedback #6(w67) -> (w110:u16)
    n113 = Subtract(x=w67, y=1) -> (x-y=→"多列列表框":i32)
    n114 = Not Equal?(x=w67, y=w110) -> (x != y?=w109:bool)
    n115 = case shown="真" w109 {
      tunnel: w67 -> [_ w259]
      tunnel: w104 -> [_ w266]
      tunnel: w103 -> [_ w265]
      frame False {
      }
      frame True {
        n116 = Subtract(x=w259, y=1) -> (x-y=w257:i32)
        n117 = Subtract(x=w257, y=5) -> (x-y=w261:i32)
        n118 = property on="多列列表框" class="MCListbox (严格)"("ItemNames"=w266, "RowHdrs[]"=w265) -> (error out=w267:errorcluster)  [unwired: 2 in, 1 out]
        n119 = Greater Or Equal To 0?(x=w261) -> (x >= 0?=w260:bool)
        n120 = property on="多列列表框" class="MCListbox (严格)"(error in=w267) -> (error out=w268:errorcluster, "TopLeft"=w269:T13)  [unwired: 1 in, 1 out]
        n121 = Select(t=w261, s=w260, f=0) -> (s? t:f=w262:i32)
        n122 = Bundle By Name(cluster=w269, "Row"=w262) -> (w270:T13)
        n123 = property on="多列列表框" class="MCListbox (严格)"(error in=w268, "TopLeft"=w270) -> ()  [unwired: 1 in, 2 out]
      }
    }
  }
  n124 = node-c288() -> (w5:T14)  [unwired: 4 in]
  n125 = property class="VI"(reference=w23) -> ("Name"=w16:string)  [unwired: 1 in, 2 out]
  n126 = control-ref of="测量模式下拉列表"() -> (w12:refnum<vi>)
  n127 = control-ref of="量程切换阈值"() -> (w10:refnum<vi>)
  n128 = control-ref of="参数下拉列表"() -> (w13:refnum<vi>)
  n129 = control-ref of="量程下拉列表"() -> (w14:refnum<vi>)
  n130 = control-ref of="备用系数"() -> (w9:refnum<vi>)
  n131 = Open VI Reference(type specifier VI Refnum (for type only)=refnum<vi> refnum, vi path=w30, options=128 ("选项")) -> (vi reference=w28:refnum<vi>, error out=w26:errorcluster)  [unwired: 3 in]
  n132 = control-ref of="公式"() -> (w11:refnum<vi>)
  n133 = timed-loop {
    timing: w5 -> [_]
    timing-out: [_] -> w4
    tunnel: w1 -> [w273]
    stop <- FALSE stop-if-true
    w274 = u16 3 items=["总磷"=1, "氨氮"=3] ("站号")
    # "定时更新"
    n134 = node-c288() -> ()  [unwired: 1 in, 1 out]
    n135 = call "总磷氨氮版本号读取.vi"() -> ("固件版本号"=→"固件版本号":string)  [unwired: 11 in]
    n136 = Bundle By Name(cluster=cluster{"命令":string, "data":variant} {"命令"="", "data"=variant} ("元素"), "命令"="读序列号", "data"=w274) -> (w272:cluster{"命令":string, "data":variant})
    n137 = Enqueue Element(queue=w273, element=w272) -> ()  [unwired: 2 in, 3 out]
    n138 = node-c288() -> ()  [unwired: 1 in, 1 out]
  }
  n139 = call-by-ref "?"(reference=w28, error in=w26) -> (reference out=w24:refnum<vi>, error out=w25:errorcluster)  [unwired: 12 in]
  n140 = Open VI Reference(type specifier VI Refnum (for type only)=refnum<vi> refnum, vi path=w16, options=128 ("选项")) -> (vi reference=w18:refnum<vi>, error out=w20:errorcluster)  [unwired: 3 in]
  n141 = call-by-ref "?"(reference=w18, error in=w20) -> (reference out=w22:refnum<vi>, error out=w21:errorcluster)  [unwired: 12 in]
  n142 = Close Reference(reference=w24, error in (no error)=w25) -> ()  [unwired: 1 out]
  n143 = while {
    tunnel: w34 -> [w283]
    shift-right: [w284] -> _
    shift-left: T5."待机" -> [w285]
    shift-right: [w281] -> _
    shift-left: u32 0 ("等待时间（毫秒）") -> [w282]
    stop <- FALSE stop-if-true
    n144 = global read "系统设置全局变量.vi" "氨氮自动测试量程配置"() -> (w280:T1)
    n145 = Wait (ms)(milliseconds to wait=u32 1000 ("等待时间（毫秒）")) -> ()  [unwired: 1 out]
    n146 = local read "定时启动"() -> (w286:bool)
    n147 = local write "氨氮自动测试量程配置"(w280) -> ()
    n148 = case shown="真" w286 {
      tunnel: w285 -> [_ w294]
      tunnel: [T5."待机" w293] -> w284
      tunnel: w283 -> [_ w292]
      tunnel: w282 -> [_ w291]
      tunnel: [_ w290] -> w281
      frame False {
      }
      frame True {
        n149 = case shown="\"氨氮测量中\"" w294 {
          tunnel: [T5."启动氨氮" w299 w306 w317 w325 w337] -> w293
          tunnel: w292 -> [_ w304 _ w323 _ _]
          tunnel: w291 -> [_ _ _ _ _ w340]
          tunnel: [_ _ _ _ _ w336] -> w290
          frame "待机", Default {
          }
          frame "启动氨氮" {
            n150 = call "总磷氨氮启动命令.vi"("参数"=T17 {"站号"=3, "量程切换"=enum."AUTO", "控制命令"=enum."启动测量", "模式设置"=enum."待机", "测量间隔"=0}) -> ("启动命令"=w297:cluster{"命令":string, "data":variant})  [unwired: 10 in]
            n151 = Enqueue Element(queue=w304, element=w297) -> ()  [unwired: 2 in, 3 out]
            n152 = global read "VAR氨氮全局变量.vi" "状态告警区"() -> (w303:T4)
            n153 = Unbundle By Name(w303) -> ("工作状态"=w302:T8)
            n154 = Not Equal To 0?(x=w302) -> (x != 0?=w301:bool)
            n155 = Select(t=T5."氨氮测量中", s=w301, f=T5."启动氨氮") -> (s? t:f=w299:T5)
          }
          frame "氨氮测量中" {
            n156 = flat-sequence {
              tunnel: [w310] -> w305
              tunnel: [w314] -> w306
              tunnel: w305 -> [w314]
              frame #0 {
                n157 = global read "VAR氨氮全局变量.vi" "状态告警区"() -> (w311:T4)
                n158 = Unbundle By Name(w311) -> ("工作状态"=w312:T8)
                n159 = Equal To 0?(x=w312) -> (x = 0?=w307:bool)
                n160 = Select(t=T5."延时", s=w307, f=T5."氨氮测量中") -> (s? t:f=w310:T5)
              }
              frame #1 {
                n161 = Wait (ms)(milliseconds to wait=u32 5000 ("等待时间（毫秒）")) -> ()  [unwired: 1 out]
              }
            }
          }
          frame "启动总磷" {
            n162 = call "总磷氨氮启动命令.vi"("参数"=T17 {"站号"=1, "量程切换"=enum."AUTO", "控制命令"=enum."启动测量", "模式设置"=enum."待机", "测量间隔"=0}) -> ("启动命令"=w316:cluster{"命令":string, "data":variant})  [unwired: 10 in]
            n163 = Enqueue Element(queue=w323, element=w316) -> ()  [unwired: 2 in, 3 out]
            n164 = global read "VAR氨氮全局变量.vi" "状态告警区"() -> (w318:T4)
            n165 = Unbundle By Name(w318) -> ("工作状态"=w319:T8)
            n166 = Not Equal To 0?(x=w319) -> (x != 0?=w320:bool)
            n167 = Select(t=T5."总磷测量中", s=w320, f=T5."启动总磷") -> (s? t:f=w317:T5)
          }
          frame "总磷测量中" {
            n168 = flat-sequence {
              tunnel: [w327] -> w324
              tunnel: [w333] -> w325
              tunnel: w324 -> [w333]
              frame #0 {
                n169 = global read "VAR氨氮全局变量.vi" "状态告警区"() -> (w330:T4)
                n170 = Unbundle By Name(w330) -> ("工作状态"=w331:T8)
                n171 = Equal To 0?(x=w331) -> (x = 0?=w326:bool)
                n172 = Select(t=T5."延时", s=w326, f=T5."总磷测量中") -> (s? t:f=w327:T5)
              }
              frame #1 {
                n173 = Wait (ms)(milliseconds to wait=u32 5000 ("等待时间（毫秒）")) -> ()  [unwired: 1 out]
              }
            }
          }
          frame "延时" {
            n174 = local read "设置值"() -> (w339:dbl)
            n175 = Increment(x=w340) -> (x+1=w336:u32)
            n176 = Greater Or Equal?(x=w336, y=w339) -> (x >= y?=w338:bool)
            n177 = Select(t=T5."待机", s=w338, f=T5."延时") -> (s? t:f=w337:T5)
          }
        }
      }
    }
  }
  n178 = while {
    tunnel: w34 -> [w347]
    tunnel: w14 -> [w346]
    tunnel: w13 -> [w345]
    tunnel: w12 -> [w344]
    tunnel: w11 -> [w343]
    tunnel: w10 -> [w342]
    tunnel: w9 -> [w341]
    tunnel: w7 -> [_]
    stop <- FALSE stop-if-true
    n179 = event shown="[10] \"读公式\": 值改变" {
      selector: _ -> [_ _ _ _ _ _ _ _ _ _ _ _ _ _ _ _]
      dyn-events: _ -> [_ _ _ _ _ _ _ _ _ _ _ _ _ _ _ _]
      timeout: _ -> [_ _ _ _ _ _ _ _ _ _ _ _ _ _ _ _]
      tunnel: w347 -> [_ _ w366 _ w377 w379 _ _ _ _ _ _ _ _ _ _]
      tunnel: w346 -> [_ _ _ _ _ _ _ _ _ _ w432 _ w452 w461 _ _]
      tunnel: w345 -> [_ _ _ _ _ _ _ _ _ _ w430 _ w450 w463 w471 w478]
      tunnel: w344 -> [_ _ _ _ _ _ _ _ _ _ w431 _ w451 w462 _ _]
      tunnel: w343 -> [_ _ _ _ _ _ _ _ _ _ w426 _ _ _ _ _]
      tunnel: w342 -> [_ _ _ _ _ _ _ _ _ _ _ _ w446 _ _ _]
      tunnel: w341 -> [_ _ _ _ _ _ _ _ _ _ _ _ _ _ w469 _]
      event Timeout {
        n180 = event-data() -> ()  [unwired: 1 in, 3 out]
      }
      event "氨氮自动测试量程配置": Value Change {
        n181 = event-data() -> ()  [unwired: 1 in, 6 out]
        n182 = flat-sequence {
          frame #0 {
            n183 = global write "系统设置全局变量.vi" "氨氮自动测试量程配置"("氨氮自动测试量程配置") -> ()
          }
          frame #1 {
            n184 = call <vilib>:"Application Directory.vi"() -> ("Application Directory"=w363:path)
            n185 = Build Path(base path=w363, name or relative path="data\\sys.ini" ("名称或相对路径")) -> (appended path=w361:path)
            n186 = vi-ref "系统设置全局变量.vi"() -> (w359:refnum<vi>)
            n187 = call <vilib>:"Open Config Data.vi"("configuration file path"=w361) -> ("error out"=w357:errorcluster, "refnum"=w360:T18)  [unwired: 8 in, 1 out]
            n188 = call <userlib>:"Write Panel to INI__ogtk.vi"("error in (no error)"=w357, "VI ref"=w359, "refnum"=w360) -> ("error out"=w356:errorcluster, "refnum out"=w358:T18)  [unwired: 7 in]
            n189 = call <vilib>:"Close Config Data.vi"("error in (no error)"=w356, "refnum"=w358) -> ("error out"=w351:errorcluster, "file path"=w350:path)  [unwired: 8 in]
            n190 = Open/Create/Replace File(file path (use dialog)=w350, error in=w351) -> (refnum out=w354:refnum<file>, error out=w355:errorcluster)  [unwired: 4 in, 1 out]
            n191 = Flush File(refnum=w354, error in=w355) -> (refnum out=w353:refnum<file>, error out=w352:errorcluster)
            n192 = Close File(refnum=w353, error in=w352) -> ()  [unwired: 2 out]
          }
        }
      }
      event "手动启动": Value Change {
        n193 = event-data() -> ()  [unwired: 1 in, 6 out]
        n194 = call "总磷氨氮启动参数对话框.vi"() -> ("确认"=w364:bool, "元素"=w365:cluster{"命令":string, "data":variant})  [unwired: 10 in]
        n195 = case shown="真" w364 {
          tunnel: w366 -> [_ w368]
          tunnel: w365 -> [_ w367]
          frame False {
          }
          frame True {
            n196 = Enqueue Element(queue=w368, element=w367) -> ()  [unwired: 2 in, 3 out]
          }
        }
      }
      event "定时启动": Mouse Down {
        n197 = event-data() -> ()  [unwired: 1 in, 6 out]
        n198 = call "定时启动对话框.vi"() -> ("设置值"=→"设置值":dbl, "确定输出"=→"定时启动":bool)  [unwired: 10 in]
      }
      event "单步测试": Value Change {
        w372 = u16 1 items=["总磷"=1, "氨氮"=3] ("站号")
        n199 = event-data() -> ()  [unwired: 1 in, 6 out]
        n200 = Bundle("站号"=w372, "总磷氨氮调试"="总磷氨氮调试") -> (w371:cluster{"站号":u16, "总磷氨氮调试":u16[]})  [unwired: 1 in]
        n201 = Bundle By Name(cluster=cluster{"命令":string, "data":variant} {"命令"="", "data"=variant} ("元素"), "命令"="debug", "data"=w371) -> (w374:cluster{"命令":string, "data":variant})
        n202 = Enqueue Element(queue=w377, element=w374) -> ()  [unwired: 2 in, 3 out]
      }
      event "停止": Value Change {
        n203 = event-data() -> ()  [unwired: 1 in, 6 out]
        n204 = Enqueue Element(queue=w379, element=cluster{"命令":string, "data":variant} {"命令"="启动", "data"=variant(cluster{"站号":u16, "控制命令输出":u16[]} {"站号"=3, "控制命令输出"=[2816]})} ("启动命令")) -> ()  [unwired: 2 in, 3 out]
      }
      event "设置": Value Change {
        n205 = event-data() -> ()  [unwired: 1 in, 6 out]
        n206 = property on="窗格" class="Pane"("Origin"=T6 {"Horizontal"=0, "Vertical"=628} ("原点")) -> ()  [unwired: 2 in, 2 out]
      }
      event "返回": Value Change {
        n207 = event-data() -> ()  [unwired: 1 in, 6 out]
        n208 = property on="窗格" class="Pane"("Origin"=T6 {"Horizontal"=0, "Vertical"=0} ("原点")) -> ()  [unwired: 2 in, 2 out]
      }
      event "标液浓度1", "测量吸光度1", "测量吸光度2", "标液浓度2", "测量吸光度3", "标液浓度3", "测量吸光度4", "标液浓度4", "测量吸光度5", "标液浓度5", "样品1启用", "样品3启用", "样品4启用", "样品5启用", "样品2启用", "模型", "method", "样品1 F0", "样品1 F1", "样品2 F1", "样品2 F0", "样品3 F1", "样品4 F0", "样品4 F1", "样品5 F1", "样品5 F0", "精度": Value Change {
        n209 = event-data() -> ()  [unwired: 1 in, 6 out]
        n210 = formula code="E=log(F0/F1);"("F0"="样品1 F0", "F1"="样品1 F1") -> ("E"=w403:dbl)
        "测量吸光度1" <- w403
        n211 = formula code="E=log(F0/F1);"("F0"="样品2 F0", "F1"="样品2 F1") -> ("E"=w400:dbl)
        "测量吸光度2" <- w400
        n212 = formula code="E=log(F0/F1);"("F0"="样品3 F0", "F1"="样品3 F1") -> ("E"=w397:dbl)
        "测量吸光度3" <- w397
        n213 = formula code="E=log(F0/F1);"("F0"="样品4 F0", "F1"="样品4 F1") -> ("E"=w394:dbl)
        "测量吸光度4" <- w394
        n214 = formula code="E=log(F0/F1);"("F0"="样品5 F0", "F1"="样品5 F1") -> ("E"=w391:dbl)
        "测量吸光度5" <- w391
        n215 = Replace Array Subset(array=dbl[] [0.0, 0.0, 0.0, 0.0, 0.0] ("数组"), new element #1="标液浓度1", new element #2="标液浓度2", new element #3="标液浓度3", new element #4="标液浓度4", new element #5="标液浓度5") -> (w388:dbl[])  [unwired: 5 in]
        n216 = Replace Array Subset(array=dbl[] [0.0, 0.0, 0.0, 0.0, 0.0] ("数组"), new element #1=w403, new element #2=w400, new element #3=w397, new element #4=w394, new element #5=w391) -> (w387:dbl[])  [unwired: 5 in]
        n217 = Replace Array Subset(array=bool[] [FALSE, FALSE, FALSE, FALSE, FALSE] ("数组"), new element #1="样品1启用", new element #2="样品2启用", new element #3="样品3启用", new element #4="样品4启用", new element #5="样品5启用") -> (w386:bool[])  [unwired: 5 in]
        n218 = call "线性公式.vi"("精度"="精度", "模型"="模型", "method"="method", "启用"=w386, "监测浓度"=w387, "标液浓度"=w388) -> ("XY图"=→"XY图":cluster{"X Values":dbl[], "Y Values":dbl[]}[], "r^2"=→"r^2":dbl, "拟合方程"=→"拟合公式":string)  [unwired: 3 in]
      }
      event "标液浓度1", "标液浓度2", "标液浓度3", "标液浓度4", "标液浓度5", "样品1 F0", "样品1 F1", "样品2 F1", "样品2 F0", "样品3 F1", "样品3 F0", "样品4 F0", "样品4 F1", "样品5 F0", "样品5 F1", "精度", "公式.X^2", "公式.X", "公式.b", "量程切换阈值.阈值", "量程切换阈值.标液浓度", "备用系数.量程上限", "备用系数.量程下限", "备用系数.检出限", "备用系数.精度": Mouse Down {
        n219 = event-data() -> ("CtlRef"=w422:refnum<vi>)  [unwired: 1 in, 5 out]
        n220 = property class="DigNum (严格)"(reference=w422) -> (reference out=w420:refnum<vi>, "Value"=w421:dbl)  [unwired: 1 in, 1 out]
        n221 = call "数字键盘.vi"("OldNumber"=w421) -> ("NewNumber"=w419:sgl)
        n222 = property class="DigNum (严格)"(reference=w420, "Val(Sgnl)"=w419) -> ()  [unwired: 1 in, 2 out]
      }
      event "读公式": Value Change {
        n223 = event-data() -> ()  [unwired: 1 in, 6 out]
        n224 = property class="Enum (严格)"(reference=w430) -> ("Value"=w429:enum16{"氨氮", "总磷"})  [unwired: 1 in, 2 out]
        n225 = property class="Enum (严格)"(reference=w431) -> ("Value"=w428:enum16{"水样测量", "空白核查", "跨度核查", "标样核查", "加标回收"})  [unwired: 1 in, 2 out]
        n226 = property class="Enum (严格)"(reference=w432) -> ("Value"=w427:enum16{"低量程", "高量程"})  [unwired: 1 in, 2 out]
        n227 = call "总磷氨氮公式读取.vi"("量程"=w427, "测量模式"=w428, "测量参数"=w429) -> ("error out"=w424:errorcluster, "公式"=w425:cluster{"X^2":dbl, "X":dbl, "b":dbl})  [unwired: 7 in]
        n228 = property class="Clust (严格)"(reference=w426, "Value"=w425) -> ()  [unwired: 1 in, 2 out]
        n229 = case shown="错误" w424 {
          tunnel: ["读取成功" ("消息") "读取失败" ("消息")] -> w423
          frame No Error {
          }
          frame Error {
          }
        }
        n230 = One Button Dialog(message=w423) -> ()  [unwired: 1 in, 1 out]
      }
      event "写公式": Value Change {
        n231 = event-data() -> ()  [unwired: 1 in, 6 out]
        n232 = call "总磷氨氮公式写入.vi"("公式"="公式", "量程"="量程下拉列表", "测量模式"="测量模式下拉列表", "测量参数"="参数下拉列表") -> ("error out"=w435:errorcluster)  [unwired: 7 in]
        n233 = case shown="无错误" w435 {
          tunnel: ["写入成功" ("消息") "写入失败" ("消息")] -> w436
          frame No Error {
          }
          frame Error {
          }
        }
        n234 = One Button Dialog(message=w436) -> ()  [unwired: 1 in, 1 out]
      }
      event "量程切换阈值读取": Value Change {
        n235 = event-data() -> ()  [unwired: 1 in, 6 out]
        n236 = property class="Enum (严格)"(reference=w450) -> ("Value"=w449:enum16{"氨氮", "总磷"})  [unwired: 1 in, 2 out]
        n237 = property class="Enum (严格)"(reference=w451) -> ("Value"=w448:enum16{"水样测量", "空白核查", "跨度核查", "标样核查", "加标回收"})  [unwired: 1 in, 2 out]
        n238 = property class="Enum (严格)"(reference=w452) -> ("Value"=w447:enum16{"低量程", "高量程"})  [unwired: 1 in, 2 out]
        n239 = call "总磷氨氮量程读取.vi"("量程"=w447, "测量模式"=w448, "测量参数"=w449) -> ("error out"=w443:errorcluster, "量程切换阈值"=w445:cluster{"阈值":dbl, "标液浓度":dbl})  [unwired: 7 in]
        n240 = property class="Clust (严格)"(reference=w446, "Value"=w445) -> ()  [unwired: 1 in, 2 out]
        n241 = case shown="错误" w443 {
          tunnel: ["读取成功" ("消息") "读取失败" ("消息")] -> w444
          frame No Error {
          }
          frame Error {
          }
        }
        n242 = One Button Dialog(message=w444) -> ()  [unwired: 1 in, 1 out]
      }
      event "量程切换阈值写入": Value Change {
        n243 = event-data() -> ()  [unwired: 1 in, 6 out]
        n244 = property class="Enum (严格)"(reference=w463) -> ("Value"=w460:enum16{"氨氮", "总磷"})  [unwired: 1 in, 2 out]
        n245 = property class="Enum (严格)"(reference=w462) -> ("Value"=w459:enum16{"水样测量", "空白核查", "跨度核查", "标样核查", "加标回收"})  [unwired: 1 in, 2 out]
        n246 = property class="Enum (严格)"(reference=w461) -> ("Value"=w458:enum16{"低量程", "高量程"})  [unwired: 1 in, 2 out]
        n247 = call "总磷氨氮量程写入.vi"("量程切换阈值"="量程切换阈值", "量程"=w458, "测量模式"=w459, "测量参数"=w460) -> ("error out"=w455:errorcluster)  [unwired: 7 in]
        n248 = case shown="无错误" w455 {
          tunnel: ["写入成功" ("消息") "写入失败" ("消息")] -> w456
          frame No Error {
          }
          frame Error {
          }
        }
        n249 = One Button Dialog(message=w456) -> ()  [unwired: 1 in, 1 out]
      }
      event "备用系数读取": Value Change {
        n250 = event-data() -> ()  [unwired: 1 in, 6 out]
        n251 = property class="Enum (严格)"(reference=w471) -> ("Value"=w470:enum16{"氨氮", "总磷"})  [unwired: 1 in, 2 out]
        n252 = call "总磷氨氮备用系数读取.vi"("测量参数"=w470) -> ("error out"=w466:errorcluster, "备用系数"=w468:T2)  [unwired: 9 in]
        n253 = property class="Clust (严格)"(reference=w469, "Value"=w468) -> ()  [unwired: 1 in, 2 out]
        n254 = case shown="错误" w466 {
          tunnel: ["读取成功" ("消息") "读取失败" ("消息")] -> w467
          frame No Error {
          }
          frame Error {
          }
        }
        n255 = One Button Dialog(message=w467) -> ()  [unwired: 1 in, 1 out]
      }
      event "备用系数写入": Value Change {
        n256 = event-data() -> ()  [unwired: 1 in, 6 out]
        n257 = property class="Enum (严格)"(reference=w478) -> ("Value"=w477:enum16{"氨氮", "总磷"})  [unwired: 1 in, 2 out]
        n258 = call "总磷氨氮备用系数写入.vi"("备用系数"="备用系数", "测量参数"=w477) -> ("error out"=w474:errorcluster)  [unwired: 9 in]
        n259 = case shown="无错误" w474 {
          tunnel: ["写入成功" ("消息") "写入失败" ("消息")] -> w475
          frame No Error {
          }
          frame Error {
          }
        }
        n260 = One Button Dialog(message=w475) -> ()  [unwired: 1 in, 1 out]
      }
    }
  }
  n261 = while {
    tunnel: w34 -> [w496]
    tunnel: w35 -> [_]
    shift-right: [w490] -> _
    shift-left: enum16{"氨氮", "总磷"}."氨氮" ("枚举") -> [w491]
    stop <- FALSE stop-if-true
    w489 = u16 3 items=["总磷"=1, "氨氮"=3] ("站号")
    # "试剂填充 172 \n管路清洗108\n氨氮92\n总磷131\n总磷海水147\n总氮76\n总氮海水92"
    n262 = Wait (ms)(milliseconds to wait=u32 1000 ("等待时间（毫秒）")) -> ()  [unwired: 1 out]
    n263 = Bundle By Name(cluster=cluster{"命令":string, "data":variant} {"命令"="", "data"=variant} ("元素"), "命令"="读状态告警区", "data"=w489) -> (w498:cluster{"命令":string, "data":variant})
    n264 = global read "VAR氨氮全局变量.vi" "状态告警区"() -> (w487:T4)
    n265 = Bundle By Name(cluster=cluster{"命令":string, "data":variant} {"命令"="", "data"=variant} ("元素"), "命令"="读测量数据区", "data"=w489) -> (w494:cluster{"命令":string, "data":variant})
    n266 = Unbundle By Name(w487) -> ("系统时间"=w486:timestamp)
    n267 = Enqueue Element(queue=w496, element=w498) -> (queue out=w492:refnum<queue>)  [unwired: 2 in, 2 out]
    n268 = Enqueue Element(queue=w492, element=w494) -> (queue out=w488:refnum<queue>)  [unwired: 2 in, 2 out]
    n269 = Get Date/Time In Seconds() -> (seconds since 1Jan1904=w485:timestamp)
    n270 = Subtract(x=w485, y=w486) -> (x-y=w484:dbl)
    n271 = Absolute Value(x=w484) -> (abs(x)=w483:dbl)
    n272 = Greater Or Equal?(x=w483, y=120.0) -> (x >= y?=w481:bool)
    n273 = case shown="真" w481 {
      tunnel: w488 -> [_ w503]
      frame False {
      }
      frame True {
        n274 = call "总磷氨氮启动命令.vi"("参数"=T19 {"站号"=3, "量程切换"=enum."AUTO", "控制命令"=enum."校时", "模式设置"=enum."待机", "测量间隔"=0}) -> ("启动命令"=w502:cluster{"命令":string, "data":variant})  [unwired: 10 in]
        n275 = Enqueue Element(queue=w503, element=w502) -> ()  [unwired: 2 in, 3 out]
      }
    }
    n276 = Increment(x=w491) -> (x+1=w490:enum16{"氨氮", "总磷"})
  }
  n277 = Close Reference(reference=w22, error in (no error)=w21) -> ()  [unwired: 1 out]
  n278 = node-c288(w4) -> ()  [unwired: 1 out]
